vi "GetURL.vi"(11 "TCP":refnum<k5>) -> (0 "reply":string, 1 "payload":string, 2 "path":T1, 3 "TCP out":refnum<k5>)   [LabVIEW 2020]
panel:
  out "size":i32
  out "Numeric":i32
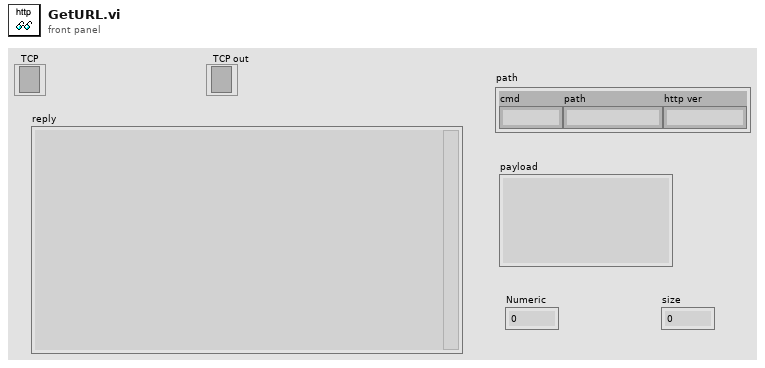
[diagram p1: front panel]
types:
  T1 = cluster{"cmd":string, "path":string, "http ver":string}
  T2 = enum16{"Standard", "Buffered", "CRLF", "Immediate"}
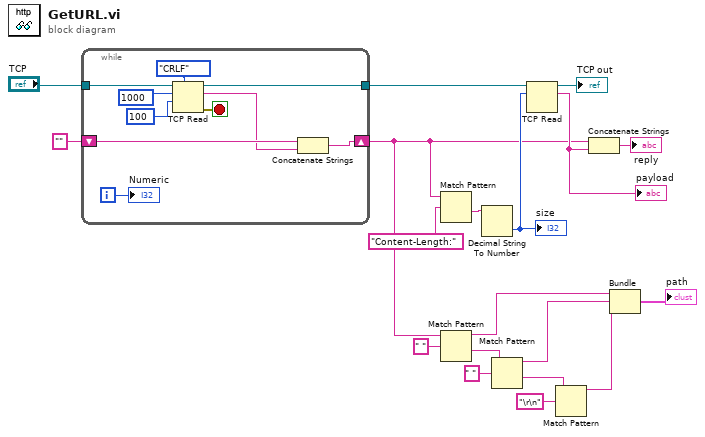
[diagram p0: block diagram]
diagram:
  n1 = while {
    tunnel: "TCP" -> [w29]
    tunnel: [w24] -> w14
    shift-right: [w21] -> w9
    shift-left: "" -> [w23]
    i -> [w25]
    stop <- w26 stop-if-true
    n2 = TCP Read(connection ID=w29, bytes to read=1000, 7:T2."CRLF" ("mode (standard)"), 9:100 ("timeout ms (25000)")) -> (connection ID out=w24:refnum<k5>, data out=w22:string, error out=w26:errorcluster)  [unwired: 1 in]
    n3 = Concatenate Strings(w23, w22) -> (w21:string)
    "Numeric" <- w25
  }
  n4 = Match Pattern(string=w9, regular expression="Content-Length:") -> (after substring=w17:string)  [unwired: 1 in, 3 out]
  n5 = Match Pattern(string=w9, regular expression=" ") -> (before substring=w4:string, after substring=w7:string)  [unwired: 1 in, 2 out]
  n6 = Decimal String To Number(string=w17) -> (number=w11:i32)  [unwired: 2 in, 1 out]
  "size" <- w11
  n7 = Match Pattern(string=w7, regular expression=" ") -> (before substring=w3:string, after substring=w5:string)  [unwired: 1 in, 2 out]
  n8 = TCP Read(connection ID=w14, bytes to read=w11) -> (connection ID out=→"TCP out":refnum<k5>, data out=w16:string)  [unwired: 3 in, 1 out]
  "payload" <- w16
  n9 = Match Pattern(string=w5, regular expression="\r\n") -> (before substring=w2:string)  [unwired: 1 in, 3 out]
  n10 = Concatenate Strings(w9, w16) -> (→"reply":string)
  n11 = Bundle(w4, w3, w2) -> (→"path":cluster{string, string, string})  [unwired: 1 in]
